vi "navX AE Example v1 .vi"() -> ()   [LabVIEW 2015]
uses:
  navX Library v2/_TypeDefs/Flags/Z900_navX_Flags_HardwareRevTypeDef.ctl
  navX Library v2/_TypeDefs/Flags/Z900_navX_Flags_OmnimountConfigTypeDef.ctl
  navX Library v2/_TypeDefs/Flags/Z900_navX_Flags_OpStatusTypeDef.ctl
  navX Library v2/_TypeDefs/Flags/Z900_navX_Flags_CalibrationStatusTypeDef.ctl
  navX AE v1/TypeDefs/FRIC_navX_DeviceNumbersTypeDef.ctl
  <vilib>/Rock Robotics/SystemInterfaces/spilib/spi_bus.ctl
  _NI WPI Serial USB/WPI_SerialPort_USB.ctl
  navX Library v2/_TypeDefs/Z900_navX_SerialStreamTypeDef.ctl
  navX AE v1/IO/Internal/Processing Loop/FRIC_navX_Internal_SPI_ProcessingLoop.vi
  navX AE v1/IO/Internal/Processing Loop/FRIC_navX_Internal_Serial_ProcessingLoop.vi
  _NI WPI Serial USB/_NI WPI Serial USB.lvlib
  navX Library v2/navX Library v2.lvlib
panel:
  in  "stop 2":bool
  out "Displacement 2":T1
  out "MPUTemp 2":dbl
  out "Board Information 2":T4 {"Board"."Hardware Revision" items=["navX-MXP"=33, "navX-Micro"=40]; "Omnimount Config" items=["DEFAULT", "X_UP", "X_DOWN", "Y_UP", "Y_DOWN", "Z_UP", "Z_DOWN"]}
  out "Linear Acceleration 2":T5
  out "Raw Values (out) 2":T6
  out "Quaternion 2":T7
  out "Status 2":T10 {"OP Status" items=["INITIALIZING", "SELFTEST_IN_PROGRESS", "ERROR", "IMU_AUTOCAL_IN_PROGRESS", "NORMAL"]; "Calibration Status" items=["IMU_CAL_STATE_MASK"=3, "IMU_CAL_STATE_INPROGRESS"=0, "IMU_CAL_STATE_ACCUMULATE"=1, "IMU_CAL_STATE_COMPLETE"=2]}
  out "YRPHfH 2":T11
  out "Timestamp 2":u32
  out "Timestamp":u32
  out "YRPHfH":T11
  out "Status":T10 {"OP Status" items=["INITIALIZING", "SELFTEST_IN_PROGRESS", "ERROR", "IMU_AUTOCAL_IN_PROGRESS", "NORMAL"]; "Calibration Status" items=["IMU_CAL_STATE_MASK"=3, "IMU_CAL_STATE_INPROGRESS"=0, "IMU_CAL_STATE_ACCUMULATE"=1, "IMU_CAL_STATE_COMPLETE"=2]}
  out "Quaternion":T7
  out "Raw Values (out)":T6
  out "Linear Acceleration":T5
  out "Board Information":T4 {"Board"."Hardware Revision" items=["navX-MXP"=33, "navX-Micro"=40]; "Omnimount Config" items=["DEFAULT", "X_UP", "X_DOWN", "Y_UP", "Y_DOWN", "Z_UP", "Z_DOWN"]}
  out "MPUTemp":dbl
  out "Displacement":T1
  in  "stop":bool
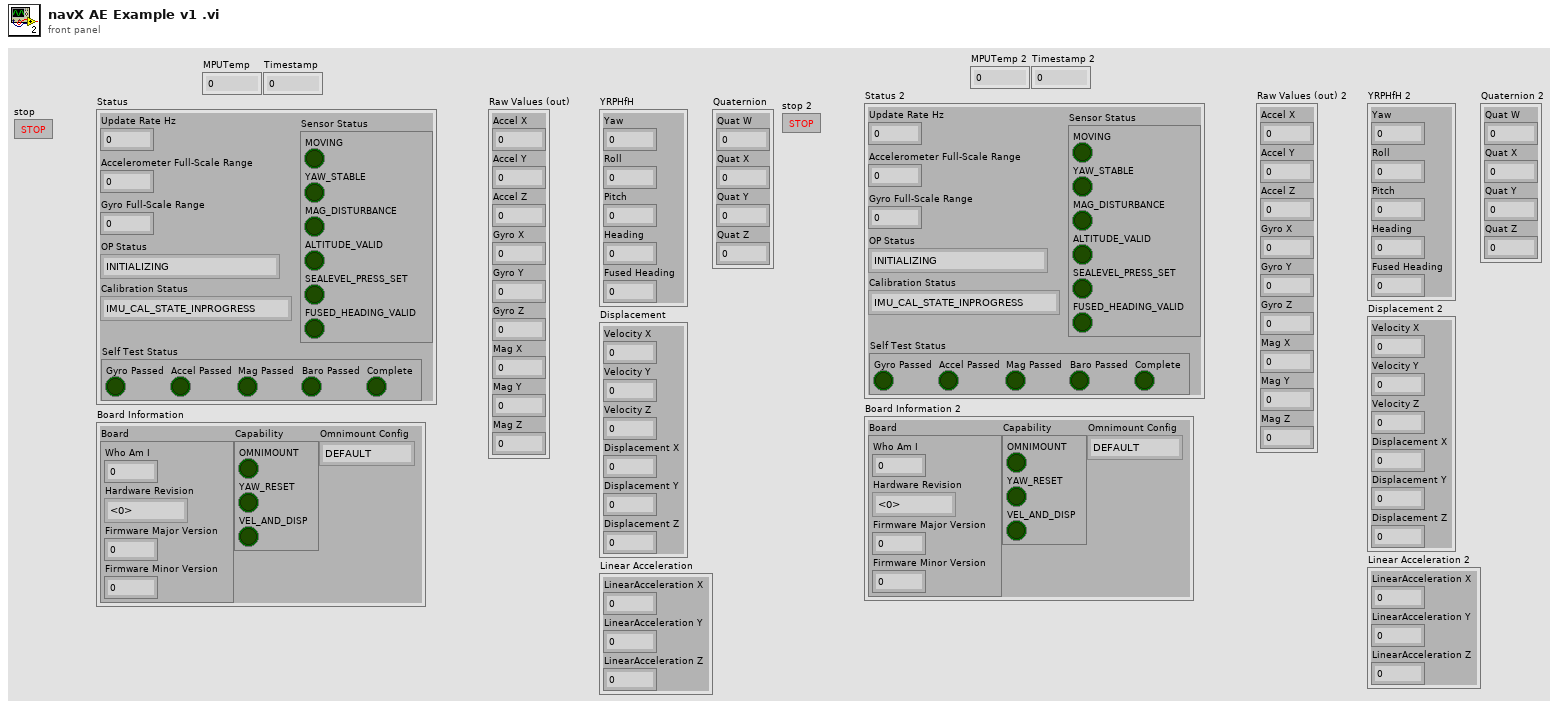
[diagram p1: front panel]
types:
  T1 = cluster{"Velocity X":dbl, "Velocity Y":dbl, "Velocity Z":dbl, "Displacement X":dbl, "Displacement Y":dbl, "Displacement Z":dbl}
  T2 = typedef "navX Library v2.lvlib/Z900_navX_Flags_HardwareRevTypeDef.ctl" = u8
  T3 = typedef "navX Library v2.lvlib/Z900_navX_Flags_OmnimountConfigTypeDef.ctl" = u8
  T4 = cluster{"Board":cluster{"Who Am I":u8, "Hardware Revision":T2, "Firmware Major Version":u8, "Firmware Minor Version":u8}, "Capability":cluster{"OMNIMOUNT":bool, "YAW_RESET":bool, "VEL_AND_DISP":bool}, "Omnimount Config":T3}
  T5 = cluster{"LinearAcceleration X":dbl, "LinearAcceleration Y":dbl, "LinearAcceleration Z":dbl}
  T6 = cluster{"Accel X":dbl, "Accel Y":dbl, "Accel Z":dbl, "Gyro X":dbl, "Gyro Y":dbl, "Gyro Z":dbl, "Mag X":dbl, "Mag Y":dbl, "Mag Z":dbl}
  T7 = cluster{"Quat W":dbl, "Quat X":dbl, "Quat Y":dbl, "Quat Z":dbl}
  T8 = typedef "navX Library v2.lvlib/Z900_navX_Flags_OpStatusTypeDef.ctl" = u8
  T9 = typedef "navX Library v2.lvlib/Z900_navX_Flags_CalibrationStatusTypeDef.ctl" = u8
  T10 = cluster{"Update Rate Hz":u8, "Accelerometer Full-Scale Range":u8, "Gyro Full-Scale Range":u16, "OP Status":T8, "Calibration Status":T9, "Sensor Status":cluster{"MOVING":bool, "YAW_STABLE":bool, "MAG_DISTURBANCE":bool, "ALTITUDE_VALID":bool, "SEALEVEL_PRESS_SET":bool, "FUSED_HEADING_VALID":bool}, "Self Test Status":cluster{"Gyro Passed":bool, "Accel Passed":bool, "Mag Passed":bool, "Baro Passed":bool, "Complete":bool}}
  T11 = cluster{"Yaw":dbl, "Roll":dbl, "Pitch":dbl, "Heading":dbl, "Fused Heading":dbl}
  T12 = typedef "navX Library v2.lvlib/Z900_navX_SerialStreamTypeDef.ctl" = enum16{"YRPH", "Quaterinons", "Gyro/Raw", "AHRS", "AHRSAndPositioning"}
  T13 = typedef "_NI WPI Serial USB.lvlib/WPI_SerialPort_USB.ctl" = enum16{"Onboard RS-232", "MXP TTL", "USB"}
  T14 = typedef "FRIC_navX_DeviceNumbersTypeDef.ctl" = enum16{"Dev0", "Dev1", "Dev2", "Dev3", "Dev4", "Dev5", "Dev6", "Dev7", "Dev8", "Dev9", "Dev10"}
  T15 = typedef "spi_bus.ctl" = enum16{"SPI On-Board, CS0", "SPI On-Board, CS1", "SPI On-Board, CS2", "SPI On-Board, CS3", "SPI MXP", "Invalid"}
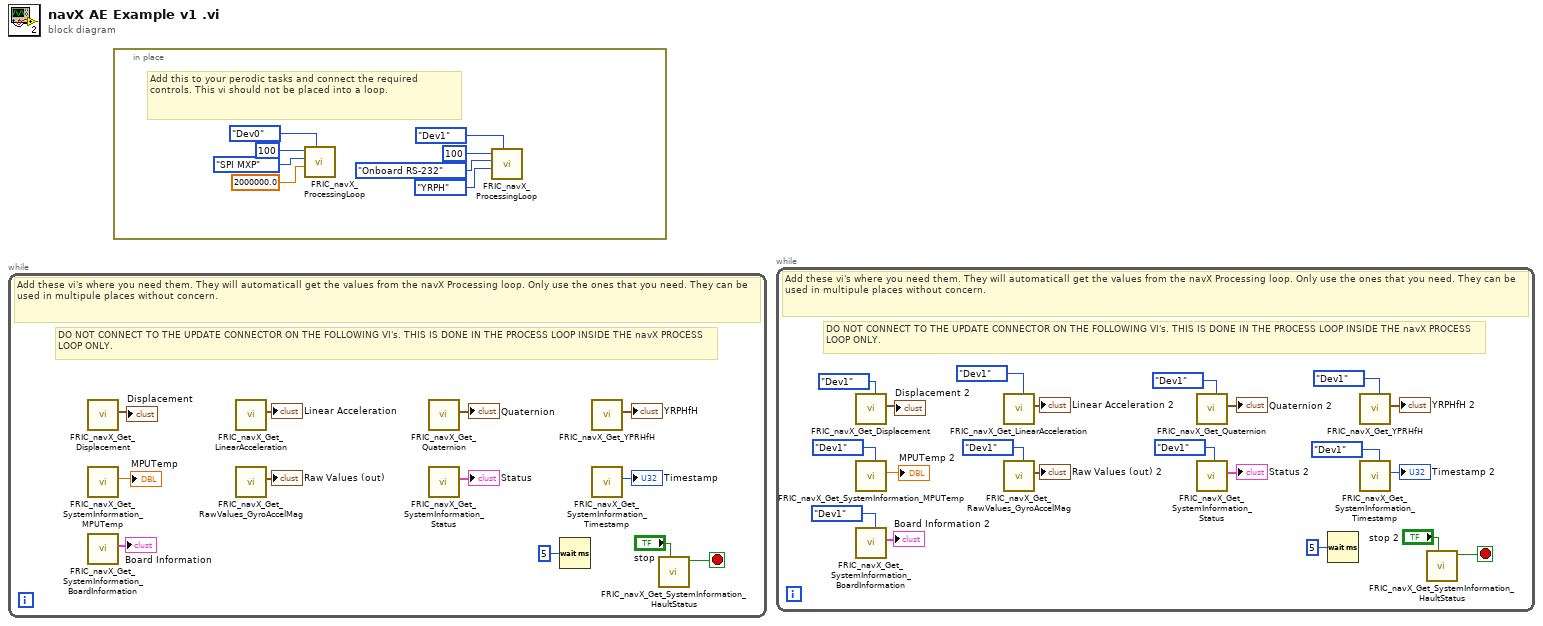
[diagram p0: block diagram]
diagram:
  n1 = while {
    stop <- w1 stop-if-true
    # "DO NOT CONNECT TO THE UPDATE CONNECTOR ON THE FOLLOWING VI's. THIS IS DONE IN THE PROCESS LOOP INSIDE THE navX PROCESS LOOP ONLY."
    # "Add these vi's where you need them. They will automaticall get the values from the navX Processing loop. Only use the ones that you need. They can be used in multipule places without concern."
    n2 = call "FRIC_navX_Get_Displacement.vi"() -> ("Displacement"=→"Displacement":T1)  [unwired: 11 in]
    n3 = call "FRIC_navX_Get_SystemInformation_MPUTemp.vi"() -> ("MPUTemp"=→"MPUTemp":dbl)  [unwired: 11 in]
    n4 = call "FRIC_navX_Get_SystemInformation_BoardInformation.vi"() -> ("Board Information"=→"Board Information":T4)  [unwired: 11 in]
    n5 = call "FRIC_navX_Get_LinearAcceleration.vi"() -> ("Linear Acceleration"=→"Linear Acceleration":T5)  [unwired: 11 in]
    n6 = call "FRIC_navX_Get_RawValues_GyroAccelMag.vi"() -> ("Raw Values (out)"=→"Raw Values (out)":T6)  [unwired: 11 in]
    n7 = call "FRIC_navX_Get_Quaternion.vi"() -> ("Quaternion"=→"Quaternion":T7)  [unwired: 11 in]
    n8 = call "FRIC_navX_Get_SystemInformation_Status.vi"() -> ("Status"=→"Status":T10)  [unwired: 11 in]
    n9 = Wait (ms)(milliseconds to wait=u32 5) -> ()  [unwired: 1 out]
    n10 = call "FRIC_navX_Get_YPRHfH.vi"() -> ("YRPHfH"=→"YRPHfH":T11)  [unwired: 11 in]
    n11 = call "FRIC_navX_Get_SystemInformation_Timestamp.vi"() -> ("Timestamp"=→"Timestamp":u32)  [unwired: 11 in]
    n12 = call "FRIC_navX_Get_SystemInformation_HaultStatus.vi"("Update"="stop") -> ("Hault"=w1:bool)  [unwired: 10 in]
  }
  n13 = in-place {
    # "Add this to your perodic tasks and connect the required controls. This vi should not be placed into a loop."
    n14 = call-poly "FRIC_navX_ProcessingLoop.vi"("Device Number"=FRIC_navX_DeviceNumbersTypeDef."Dev0", "Clock Rate (Hz)"=2000000.0, "SPI Bus"=spi_bus."SPI MXP", "Update Rate (4Hz-100Hz)"=u8 100) -> ()  [unwired: 8 in]
    n15 = call-poly "FRIC_navX_ProcessingLoop.vi"("Device Number"=FRIC_navX_DeviceNumbersTypeDef."Dev1", "Stream Type"=Z900_navX_SerialStreamTypeDef."YRPH", "Serial Port"=WPI_SerialPort_USB."Onboard RS-232", "Update Rate (4Hz-100Hz)"=u8 100) -> ()  [unwired: 8 in]
  }
  n16 = while {
    stop <- w30 stop-if-true
    # "DO NOT CONNECT TO THE UPDATE CONNECTOR ON THE FOLLOWING VI's. THIS IS DONE IN THE PROCESS LOOP INSIDE THE navX PROCESS LOOP ONLY."
    # "Add these vi's where you need them. They will automaticall get the values from the navX Processing loop. Only use the ones that you need. They can be used in multipule places without concern."
    n17 = call "FRIC_navX_Get_Displacement.vi"("Device Number"=FRIC_navX_DeviceNumbersTypeDef."Dev1") -> ("Displacement"=→"Displacement 2":T1)  [unwired: 10 in]
    n18 = call "FRIC_navX_Get_SystemInformation_MPUTemp.vi"("Device Number"=FRIC_navX_DeviceNumbersTypeDef."Dev1") -> ("MPUTemp"=→"MPUTemp 2":dbl)  [unwired: 10 in]
    n19 = call "FRIC_navX_Get_SystemInformation_BoardInformation.vi"("Device Number"=FRIC_navX_DeviceNumbersTypeDef."Dev1") -> ("Board Information"=→"Board Information 2":T4)  [unwired: 10 in]
    n20 = call "FRIC_navX_Get_LinearAcceleration.vi"("Device Number"=FRIC_navX_DeviceNumbersTypeDef."Dev1") -> ("Linear Acceleration"=→"Linear Acceleration 2":T5)  [unwired: 10 in]
    n21 = call "FRIC_navX_Get_RawValues_GyroAccelMag.vi"("Device Number"=FRIC_navX_DeviceNumbersTypeDef."Dev1") -> ("Raw Values (out)"=→"Raw Values (out) 2":T6)  [unwired: 10 in]
    n22 = call "FRIC_navX_Get_Quaternion.vi"("Device Number"=FRIC_navX_DeviceNumbersTypeDef."Dev1") -> ("Quaternion"=→"Quaternion 2":T7)  [unwired: 10 in]
    n23 = call "FRIC_navX_Get_SystemInformation_Status.vi"("Device Number"=FRIC_navX_DeviceNumbersTypeDef."Dev1") -> ("Status"=→"Status 2":T10)  [unwired: 10 in]
    n24 = Wait (ms)(milliseconds to wait=u32 5) -> ()  [unwired: 1 out]
    n25 = call "FRIC_navX_Get_YPRHfH.vi"("Device Number"=FRIC_navX_DeviceNumbersTypeDef."Dev1") -> ("YRPHfH"=→"YRPHfH 2":T11)  [unwired: 10 in]
    n26 = call "FRIC_navX_Get_SystemInformation_Timestamp.vi"("Device Number"=FRIC_navX_DeviceNumbersTypeDef."Dev1") -> ("Timestamp"=→"Timestamp 2":u32)  [unwired: 10 in]
    n27 = call "FRIC_navX_Get_SystemInformation_HaultStatus.vi"("Update"="stop 2") -> ("Hault"=w30:bool)  [unwired: 10 in]
  }
